vi "WriteToDb.vi"(0 "reference in":refnum<class "Sig_Digital.lvclass">, 11 "error in (no error)":errorcluster) -> (4 "reference out":refnum<class "Sig_Digital.lvclass">, 15 "error out":errorcluster)   [LabVIEW 2019, in "Sig_Digital.lvclass"]
uses:
  Sig_Digital.lvclass
  D:/GIT H4000/H4000/src/Proccess_class/Proccess.lvclass
  Proccess_class/Proccess.lvclass/Proccess.ctl
  Sig_Digital.lvclass/Sig_Digital.ctl
  Logger_class/Priority.ctl
  Logger_class/EventData.ctl
  Logger_class/EventCode.ctl
  Logger_class/Logger.lvclass
  Proccess_class/Proccess.lvclass
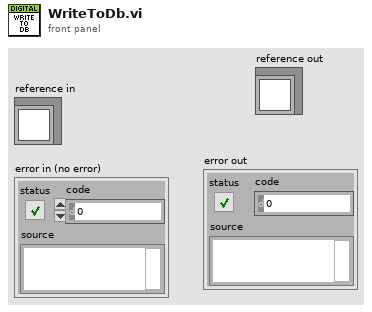
[diagram p1: front panel]
types:
  T1 = typedef "Logger.lvclass/Priority.ctl" = enum16{"Alert", "Critical", "Error", "Warning", "Notice", "Informational", "Debug"}
  T2 = typedef "Logger.lvclass/EventCode.ctl" = enum16{"DI_EU_LO", "DI_EU_HI", "DIO_LO", "DIO_HI", "DI_RAW_LO", "DI_RAW_HI", "DO_LO", "DO_HI", "DA_OK", "DA_ALARM", "AA_HI", "AA_HIHI", "AA_LO", "AA_LOLO", "AA_OK", "CMD", "OUT_OF_RANGE_OK", "OUT_OF_RANGE_LO", "OUT_OF_RANGE_HI", "CONFIG", "DI_LO", "DI_HI"}
  T3 = typedef "Logger.lvclass/EventData.ctl" = cluster{"obj_tag":string, "event_tag":string, "code":T2, "Priority":T1, "Value":dbl, "Description":string, "Time Stamp":timestamp}
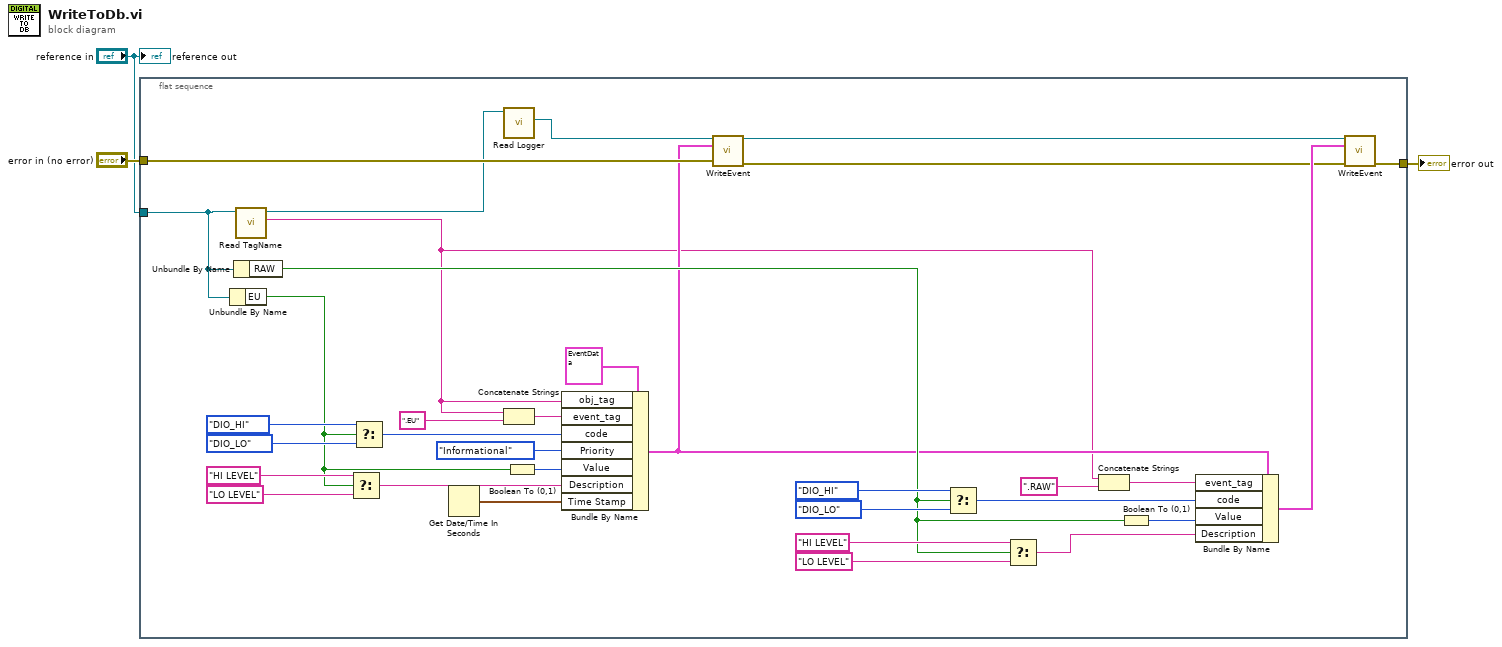
[diagram p0: block diagram]
diagram:
  n1 = flat-sequence {
    tunnel: "error in (no error)" -> [w16]
    tunnel: "reference in" -> [w5]
    tunnel: [w8] -> w3
    frame #0 {
      n2 = Unbundle By Name(w5) -> ("EU"=w13:bool)
      n3 = Unbundle By Name(w5) -> ("RAW"=w28:bool)
      n4 = call "Read TagName.vi"("Proccess in"=w5) -> ("TagName"=w6:string, "Proccess out"=w4:refnum<class "Sig_Digital.lvclass">)  [unwired: 9 in]
      n5 = Select(t="HI LEVEL" ("Description"), s=w13, f="LO LEVEL" ("Description")) -> (s? t:f=w12:string)
      n6 = Select(t=EventCode."DIO_HI" ("code"), s=w13, f=EventCode."DIO_LO" ("code")) -> (s? t:f=w20:T2)
      n7 = Get Date/Time In Seconds() -> (seconds since 1Jan1904=w17:timestamp)
      n8 = call "Read Logger.vi"("Proccess in"=w4) -> ("Logger"=w7:refnum<class "Logger.lvclass">)  [unwired: 9 in, 1 out]
      n9 = Concatenate Strings(w6, ".EU" ("string")) -> (w23:string)
      n10 = Boolean To (0,1)(Boolean=w13) -> (0, 1=w18:i16)
      n11 = Bundle By Name(cluster=T3 {"obj_tag"="", "event_tag"="", "code"=enum."DI_RAW_LO", "Priority"=enum."Alert", "Value"=0.0, "Description"="", "Time Stamp"=timestamp(0 s since 1904-01-01)} ("Event"), "obj_tag"=w6, "event_tag"=w23, "code"=w20, "Priority"=Priority."Informational", "Value"=w18, "Description"=w12, "Time Stamp"=w17) -> (w10:T3)
      n12 = call "WriteEvent.vi"("reference in"=w7, "Event"=w10, "error in (no error)"=w16) -> ("reference out"=w11:refnum<class "Logger.lvclass">, "error out"=w9:errorcluster)  [unwired: 11 in]
      n13 = Select(t=EventCode."DIO_HI" ("code"), s=w28, f=EventCode."DIO_LO" ("code")) -> (s? t:f=w31:T2)
      n14 = Select(t="HI LEVEL" ("Description"), s=w28, f="LO LEVEL" ("Description")) -> (s? t:f=w26:string)
      n15 = Concatenate Strings(w6, ".RAW" ("string")) -> (w34:string)
      n16 = Boolean To (0,1)(Boolean=w28) -> (0, 1=w30:i16)
      n17 = Bundle By Name(cluster=w10, "event_tag"=w34, "code"=w31, "Value"=w30, "Description"=w26) -> (w36:T3)
      n18 = call "WriteEvent.vi"("reference in"=w11, "Event"=w36, "error in (no error)"=w9) -> ("error out"=w8:errorcluster)  [unwired: 11 in, 1 out]
    }
  }
  "error out" <- w3
  "reference out" <- "reference in"
